vi "Write History Size.vi"(8 "error in (no error)":errorcluster, 10 "HistorySize":u32, 11 "StatusHistory in":refnum<class "StatusHistory.lvclass">) -> (0 "error out":errorcluster, 3 "StatusHistory out":refnum<class "StatusHistory.lvclass">)   [LabVIEW 2015, in "StatusHistory.lvclass"]
doc: "This property gets or sets the History Size. This is the amount of items that will be stored in the history and drawn to the string control. This also affects how many steps there are between the Most Recent Color and the Least Recent Color.\n<b> </b> <b> </b>\n©2016 Q Software Innovations, LLC (QSI)\nwritten by Quentin Alldredge\nproduced in LabVIEW 2015\n\nsupport@qsoftwareinnovations.com\nwww.qsoftwareinnovations.com\n\nAll rights reserved.\n\nRedistribution and use in source and binary forms, with or without modification, are permitted provided that the following conditions are met:\n\n * Redistributions of source code must retain the above copyright notice, this list of conditions and the following disclaimer.\n * Redistributions in binary form must reproduce the above copyright notice, this list of conditions and the following disclaimer in the documentation and/or other materials provided with the distribution.\n * Neither the name of Q Software Innovations, LLC. nor the names of its contributors may be used to endorse or promote products derived from this software without specific prior written permission.\n\nTHIS SOFTWARE IS PROVIDED BY THE COPYRIGHT HOLDERS AND CONTRIBUTORS \"AS IS\" AND ANY EXPRESS OR IMPLIED WARRANTIES, INCLUDING, BUT NOT LIMITED TO, THE IMPLIED WARRANTIES OF MERCHANTABILITY AND FITNESS FOR A PARTICULAR PURPOSE ARE DISCLAIMED. IN NO EVENT SHALL THE COPYRIGHT OWNER OR CONTRIBUTORS BE LIABLE FOR ANY DIRECT, INDIRECT, INCIDENTAL, SPECIAL, EXEMPLARY, OR CONSEQUENTIAL DAMAGES (INCLUDING, BUT NOT LIMITED TO, PROCUREMENT OF SUBSTITUTE GOODS OR SERVICES; LOSS OF USE, DATA, OR PROFITS; OR BUSINESS INTERRUPTION) HOWEVER CAUSED AND ON ANY THEORY OF LIABILITY, WHETHER IN CONTRACT, STRICT LIABILITY, OR TORT (INCLUDING NEGLIGENCE OR OTHERWISE) ARISING IN ANY WAY OUT OF THE USE OF THIS SOFTWARE, EVEN IF ADVISED OF THE POSSIBILITY OF SUCH DAMAGE."
uses:
  StatusHistory.lvclass
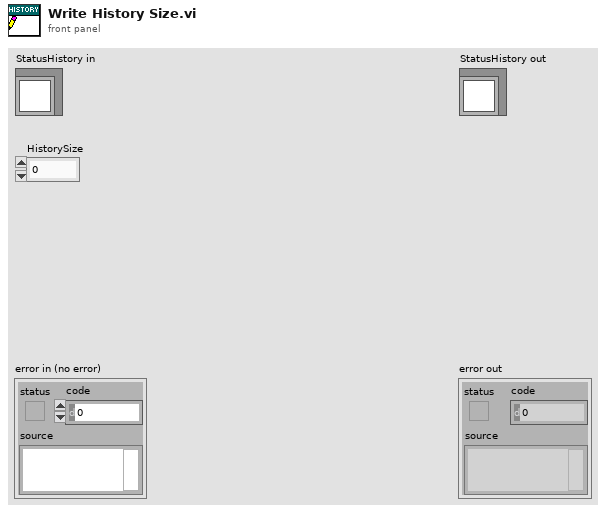
[diagram p1: front panel]
types:
  T1 = typedef "StatusHistory.lvclass/State Data.ctl" = cluster{"HistorySize":u32, "Most Recent Color":u32, "Least Recent Color":u32, "Direction":T2, "LockScrolling?":bool}
  T2 = typedef "StatusHistory.lvclass/Direction.ctl" = enum16{"Descending", "Ascending"}
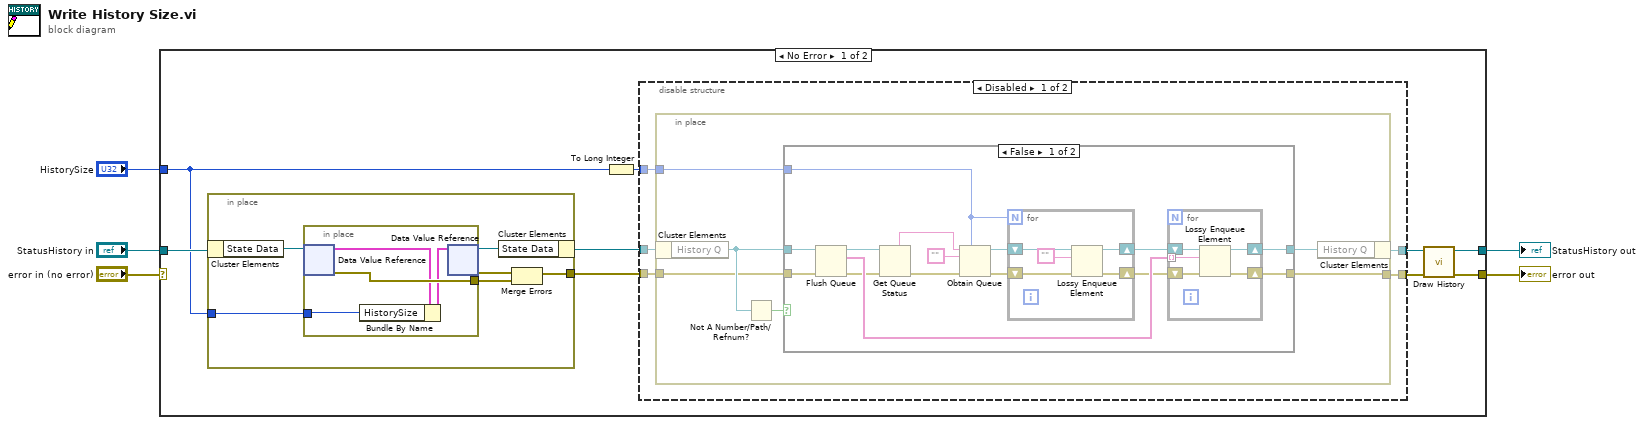
[diagram p0: block diagram]
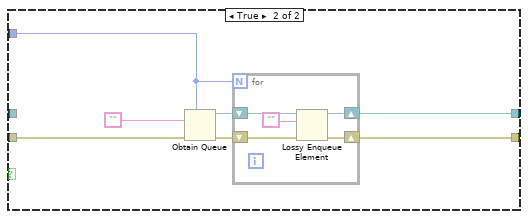
[diagram p2: hidden frame]
diagram:
  n1 = case shown="No Error" "error in (no error)" {
    selector: "error in (no error)" -> [_ w75]
    tunnel: [w12 w75] -> w4
    tunnel: [w10 w76] -> w2
    tunnel: "StatusHistory in" -> [w9 w76]
    tunnel: "HistorySize" -> [w7 _]
    frame No Error {
      n2 = in-place {
        in-place-border: [w66] -> w6
        in-place-border: w7 -> [w65]
        n3 = in-place-cluster #1(w9) -> ("State Data"=w70:refnum<data-value>)
        n4 = in-place {
          in-place-border: [w74] -> w67
          in-place-border: w65 -> [w72]
          n5 = in-place-dvr #2(w70) -> (w71:T1, w74:errorcluster)
          n6 = Bundle By Name(cluster=w71, "HistorySize"=w72) -> (w73:T1)
          n7 = in-place-dvr #2(w73) -> (w69:refnum<data-value>, w68:errorcluster)
        }
        n8 = in-place-cluster #1("State Data"=w69) -> (w8:refnum<class "StatusHistory.lvclass">)
        n9 = Merge Errors(w68, w67) -> (w66:errorcluster)
      }
      n10 = To Long Integer(number=w7) -> (32bit integer=w14:i32)
      n11 = disable-structure shown="Disabled" {
        disable-tunnel: w14 -> [w19 _]
        disable-tunnel: [w18 w63] -> w13
        disable-tunnel: [w17 w64] -> w11
        disable-tunnel: w8 -> [w16 w64]
        disable-tunnel: w6 -> [w15 w63]
        frame Disabled {
          n12 = in-place {
            in-place-border: w19 -> [w25]
            in-place-border: [w23] -> w18
            in-place-border: w15 -> [w20]
            n13 = in-place-cluster #3(w16) -> ("History Q"=w22:refnum<queue>)
            n14 = Not A Number/Path/Refnum?(number/path/refnum=w22) -> (NaN/Path/Refnum?=w21:bool)
            n15 = case shown="False" w21 {
              tunnel: w25 -> [w34 w55]
              tunnel: [w38 w53] -> w24
              tunnel: [w37 w51] -> w23
              tunnel: w22 -> [w36 _]
              tunnel: w20 -> [w35 w57]
              frame False {
                n16 = Flush Queue(queue=w36, error in (no error)=w35) -> (queue out=w26:refnum<queue>, remaining elements=w39:string[], error out=w29:errorcluster)
                n17 = Get Queue Status(queue=w26, error in (no error)=w29) -> (queue name=w27:string, error out=w28:errorcluster)  [unwired: 1 in, 6 out]
                n18 = Obtain Queue(max queue size (-1, unlimited)=w34, name (unnamed)=w27, element data type="", error in (no error)=w28) -> (queue out=w33:refnum<queue>, error out=w31:errorcluster)  [unwired: 1 in, 1 out]
                n19 = for {
                  N: w34 -> [_]
                  shift-right: [w44] -> w30
                  shift-left: w31 -> [w45]
                  shift-right: [w42] -> w32
                  shift-left: w33 -> [w43]
                  n20 = Lossy Enqueue Element(queue=w43, element="", error in (no error)=w45) -> (queue out=w42:refnum<queue>, error out=w44:errorcluster)  [unwired: 2 out]
                }
                n21 = for {
                  shift-right: [w49] -> w37
                  shift-left: w30 -> [w50]
                  tunnel: w39 -> [w48] mode=indexing
                  shift-right: [w46] -> w38
                  shift-left: w32 -> [w47]
                  n22 = Lossy Enqueue Element(queue=w47, element=w48, error in (no error)=w50) -> (queue out=w46:refnum<queue>, error out=w49:errorcluster)  [unwired: 2 out]
                }
              }
              frame True {
                n23 = Obtain Queue(max queue size (-1, unlimited)=w55, element data type="", error in (no error)=w57) -> (queue out=w54:refnum<queue>, error out=w52:errorcluster)  [unwired: 2 in, 1 out]
                n24 = for {
                  N: w55 -> [_]
                  shift-right: [w61] -> w51
                  shift-left: w52 -> [w62]
                  shift-right: [w59] -> w53
                  shift-left: w54 -> [w60]
                  n25 = Lossy Enqueue Element(queue=w60, element="", error in (no error)=w62) -> (queue out=w59:refnum<queue>, error out=w61:errorcluster)  [unwired: 2 out]
                }
              }
            }
            n26 = in-place-cluster #3("History Q"=w24) -> (w17:refnum<class "StatusHistory.lvclass">)
          }
        }
        frame Enabled {
        }
      }
      n27 = call "Draw History.vi"("error in (no error)"=w13, "StatusHistory in"=w11) -> ("error out"=w12:errorcluster, "StatusHistory out"=w10:refnum<class "StatusHistory.lvclass">)  [unwired: 8 in]
    }
    frame Error {
    }
  }
  "error out" <- w4
  "StatusHistory out" <- w2
